vi "diode_curve.vi"() -> ()   [LabVIEW 2017]
panel:
  out "Waveform Graph":dbl[](graph)
  out "Current(mA)":dbl
  out "Voltage(V)":dbl
  out "DIODE VI CHARACTERISTICS":cluster{"Y":dbl[], "Y":dbl[]}[](graph)
  in  "stop":bool
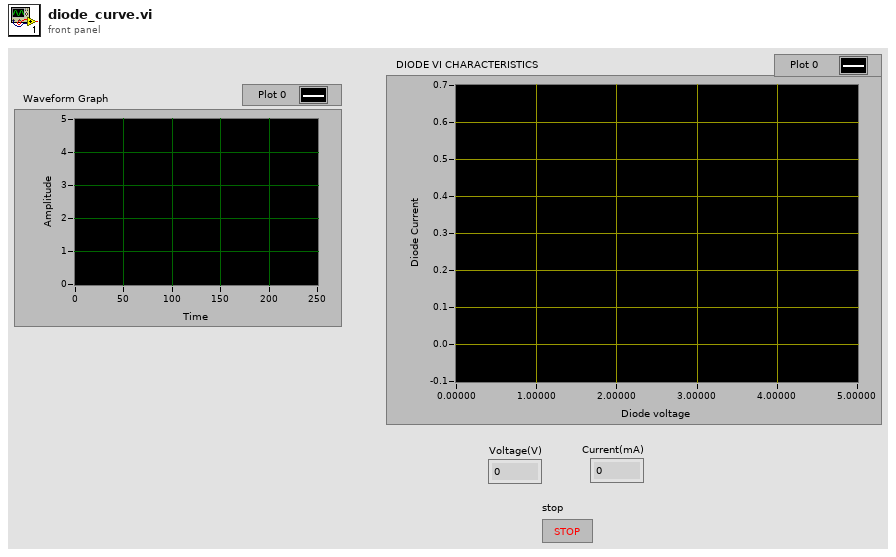
[diagram p1: front panel]
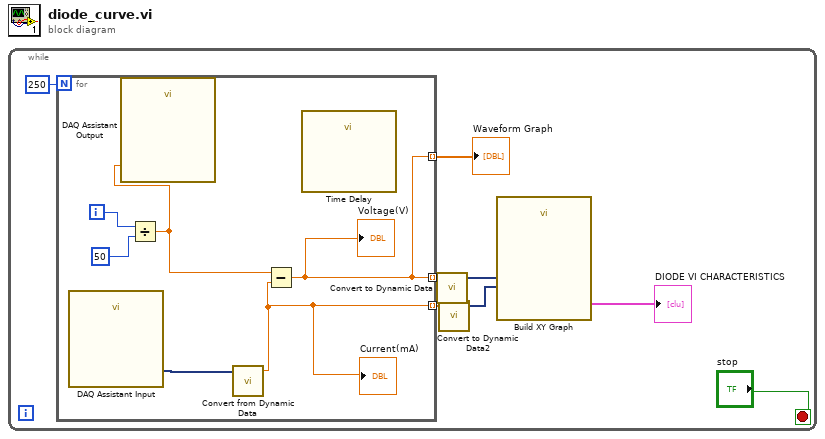
[diagram p0: block diagram]
diagram:
  n1 = while {
    stop <- "stop" stop-if-true
    n2 = for {
      N: 250 -> [_]
      tunnel: [w9] -> w7 mode=indexing
      tunnel: [w10] -> w4 mode=indexing
      tunnel: [w9] -> w1 mode=indexing
      i -> [w14]
      n3 = call "DAQ Assistant Input"() -> ("data"=w11:dynamicdata)  [unwired: 17 in, 2 out]
      n4 = Divide(x=w14, y=50) -> (x/y=w12:dbl)
      n5 = call "DAQ Assistant Output"("data"=w12) -> ()  [unwired: 17 in, 2 out]
      n6 = call "Convert from Dynamic Data"("Dynamic Data Type"=w11) -> ("Scalar"=w10:dbl)  [unwired: 3 in]
      "Current(mA)" <- w10
      n7 = Subtract(x=w12, y=w10) -> (x-y=w9:dbl)
      "Voltage(V)" <- w9
      n8 = call "Time Delay"() -> ()  [unwired: 11 in, 1 out]
    }
    "Waveform Graph" <- w1
    n9 = call "Convert to Dynamic Data"("Array"=w7) -> ("Dynamic Data Type"=w6:dynamicdata)  [unwired: 3 in]
    n10 = call "Convert to Dynamic Data2"("Array"=w4) -> ("Dynamic Data Type"=w5:dynamicdata)  [unwired: 3 in]
    n11 = call "Build XY Graph"("Y Input"=w5, "X Input"=w6) -> ("XY Graph"=→"DIODE VI CHARACTERISTICS":cluster{"X":dbl[], "Y":dbl[]}[])  [unwired: 8 in, 1 out]
  }
